vi "SigSyn (G3)-Plot.vi"(0 "Array":dbl[][](array[numeric]), 2 "Waveform Graph":refnum<vi>, 5 "Active Endpoints":string[](array[string]), 9 "Sampling Rate (Hz)":dbl, 11 "error in (no error)":errorcluster, 12 "Endpoint Config":T1[](array[typedef]), 13 "Normalize":bool) -> (4 "Array thru":dbl[][](array[numeric]), 15 "error out":errorcluster)   [LabVIEW 2020]
doc: "Helper function to plot stimuli in a sensible fashion."
uses:
  Calibration VIs/Endpoint VIs/LV Source/Endpoint-Spec.ctl
  Calibration VIs/Endpoint VIs/LV Source/Endpoint-Modality.ctl
  Calibration VIs/Endpoint VIs/LV Source/Endpoint-Laterality.ctl
  Utility VIs/Math VIs/LinSpace (x0-dx-npts).vi
  PXI DAQ VIs/Utility VIs/Array Dimensions (2D).vi
panel:
  in  "Vmax":dbl=10.0
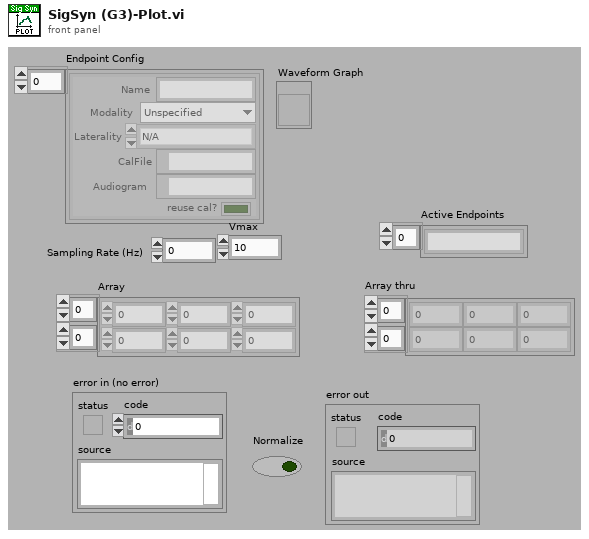
[diagram p1: front panel]
types:
  T1 = typedef "Endpoint-Spec.ctl" = cluster{"Name":string, "Modality":T2, "Laterality":T3, "CalFile":path, "Audiogram":path, "reuse cal?":bool}
  T2 = typedef "Endpoint-Modality.ctl" = enum16{"Unspecified", "Acoustic", "Electric", "Optical"}
  T3 = typedef "Endpoint-Laterality.ctl" = enum16{"N/A", "Right", "Left"}
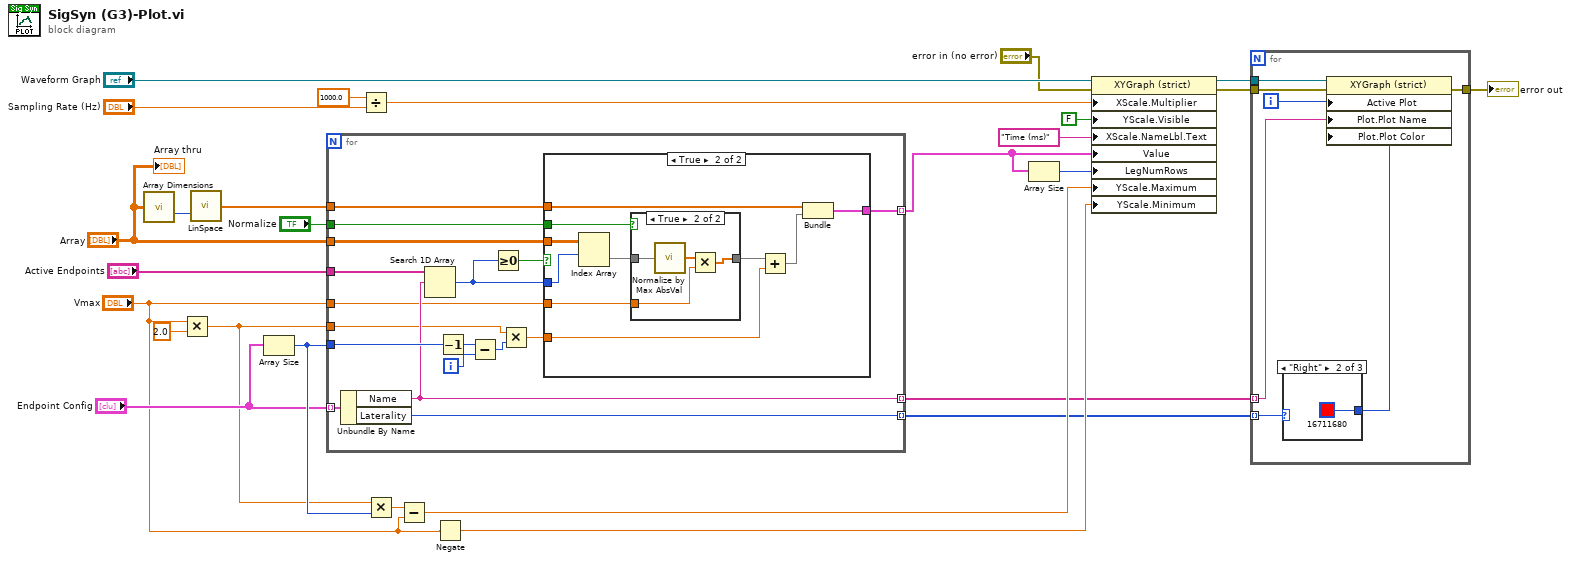
[diagram p0: block diagram]
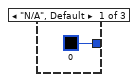
[diagram p2: hidden frame]
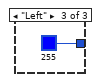
[diagram p3: hidden frame]
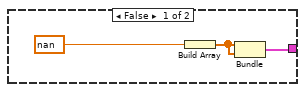
[diagram p4: hidden frame]
diagram:
  n1 = call-poly "Array Dimensions.vi"("2D Array"="Array") -> ("# columns"=w17:i32)  [unwired: 13 in, 1 out]
  n2 = Multiply(x="Vmax", y=2.0) -> (x*y=w13:dbl)
  n3 = call-poly "LinSpace.vi"("npts"=w17) -> ("Array"=w15:dbl[])  [unwired: 3 in, 1 out]
  n4 = Array Size(array="Endpoint Config") -> (size(s)=w21:i32)
  n5 = for {
    tunnel: "Endpoint Config" -> [w44] mode=indexing
    tunnel: "Array" -> [w35]
    tunnel: w21 -> [w43]
    tunnel: [w38] -> w5 mode=indexing
    tunnel: "Active Endpoints" -> [w39]
    tunnel: w15 -> [w33]
    tunnel: [w32] -> w11 mode=indexing
    tunnel: w13 -> [w31]
    tunnel: "Normalize" -> [w30]
    tunnel: "Vmax" -> [w29]
    tunnel: [w28] -> w1 mode=indexing
    i -> [w42]
    n6 = Unbundle By Name(w44) -> ("Name"=w38:string, "Laterality"=w28:T3)
    n7 = Search 1D Array(1D array=w39, element=w38) -> (index of element=w36:i32)  [unwired: 1 in]
    n8 = Decrement(x=w43) -> (x-1=w40:i32)
    n9 = Subtract(x=w40, y=w42) -> (x-y=w41:i32)
    n10 = Greater Or Equal To 0?(x=w36) -> (x >= 0?=w37:bool)
    n11 = Multiply(x=w31, y=w41) -> (x*y=w34:dbl)
    n12 = case shown="True" w37 {
      tunnel: w36 -> [_ w56]
      tunnel: w35 -> [_ w57]
      tunnel: w34 -> [_ w55]
      tunnel: w33 -> [_ w54]
      tunnel: [w47 w52] -> w32
      tunnel: w30 -> [_ w50]
      tunnel: w29 -> [_ w48]
      frame False {
        n13 = Build Array(nan) -> (w45:dbl[])
        n14 = Bundle(w45, w45) -> (w47:cluster{dbl[], dbl[]})  [unwired: 1 in]
      }
      frame True {
        n15 = Index Array(array=w57, index (row)=w56) -> (element=w51:dbl[])  [unwired: 1 in]
        n16 = case shown="True" w50 {
          tunnel: w51 -> [w58 w62]
          tunnel: [w58 w60] -> w49
          tunnel: w48 -> [_ w59]
          frame False {
          }
          frame True {
            n17 = call "Normalize by Max AbsVal.vi"("Y"=w62) -> ("Ynorm"=w61:dbl[])
            n18 = Multiply(x=w61, y=w59) -> (x*y=w60:dbl[])
          }
        }
        n19 = Add(x=w49, y=w55) -> (x+y=w53:dbl[])
        n20 = Bundle("Array"=w54, w53) -> (w52:cluster{"Array":dbl[], dbl[]})  [unwired: 1 in]
      }
    }
  }
  n21 = Divide(x=1000.0, y="Sampling Rate (Hz)") -> (x/y=w19:dbl)
  n22 = Multiply(x=w13, y=w21) -> (x*y=w20:dbl)
  n23 = Subtract(x=w20, y="Vmax") -> (x-y=w10:dbl)
  n24 = Negate(x="Vmax") -> (-x=w9:dbl)
  n25 = Array Size(array=w11) -> (size(s)=w12:i32)
  n26 = property class="XYGraph (strict)"(reference="Waveform Graph", error in="error in (no error)", "XScale.Multiplier"=w19, "YScale.Visible"=FALSE ("Y Scale.Name Label.Visible"), "XScale.NameLbl.Text"="Time (ms)" ("X Scale.Name Label.Text"), "Value"=w11, "LegNumRows"=w12, "YScale.Maximum"=w10, "YScale.Minimum"=w9) -> (reference out=w8:refnum<vi>, error out=w7:errorcluster)
  n27 = for {
    tunnel: w8 -> [w69]
    tunnel: w7 -> [w68]
    tunnel: [w67] -> w6
    tunnel: w5 -> [w65] mode=indexing
    tunnel: w1 -> [w64] mode=indexing
    i -> [w66]
    n28 = case shown="\"Right\"" w64 {
      tunnel: [u32 0 u32 16711680 u32 255] -> w63
      frame "N/A", Default {
      }
      frame "Right" {
      }
      frame "Left" {
      }
    }
    n29 = property class="XYGraph (strict)"(reference=w69, error in=w68, "Active Plot"=w66, "Plot.Plot Name"=w65, "Plot.Plot Color"=w63) -> (error out=w67:errorcluster)  [unwired: 1 out]
  }
  "error out" <- w6
  "Array thru" <- "Array"
